vi "Tab.Set.vi"(8 "error in (no error)":errorcluster, 11 "State Variables":T1) -> (0 "error out":errorcluster, 3 "State Variables out":T1)   [LabVIEW 2015]
uses:
  Types/Main.StateVariables.ctl
  <vilib>/Utility/miscctls.llb/LVPositionTypeDef.ctl
  Types/Execute.UserEventRefs.ctl
  <vilib>/NI Veristand/Execution/Workspace/SystemStateRegEventRef.ctl
  <vilib>/NI Veristand/Execution/Workspace/Target State Info.ctl
  <vilib>/NI Veristand/Execution/Workspace/Target State.ctl
  <vilib>/NI Veristand/Execution/WaveformStreaming/Waveform Data Watcher Event Data (DBL).ctl
  <vilib>/NI Veristand/Execution/WaveformStreaming/WaveformStreamSpecification.ctl
  NationalInstruments.VeriStand.ClientAPI
  <vilib>/NI Veristand/Execution/Workspace/SystemStateEventRef.ctl
  <vilib>/NI Veristand/Execution/Workspace/WorkspaceAPI.ctl
  Types/UI.Object.ctl
  Types/Waveforms.Info.ctl
  <vilib>/NI Veristand/Execution/WaveformStreaming/Registered Waveform Streams Data Event Refnum (DBL).ctl
  <vilib>/NI Veristand/Execution/WaveformStreaming/WaveformDataWatcherDBL.ctl
  <vilib>/NI Veristand/Execution/WaveformStreaming/WaveformStreamingAPI.ctl
  <vilib>/Utility/miscctls.llb/LVRowAndColumnTypeDef.ctl
  <vilib>/NI Veristand/Execution/Workspace/NI_VS Workspace ExecutionAPI.lvlib
  <vilib>/NI Veristand/Execution/WaveformStreaming/NI_VS Waveform Streaming Interface.lvlib
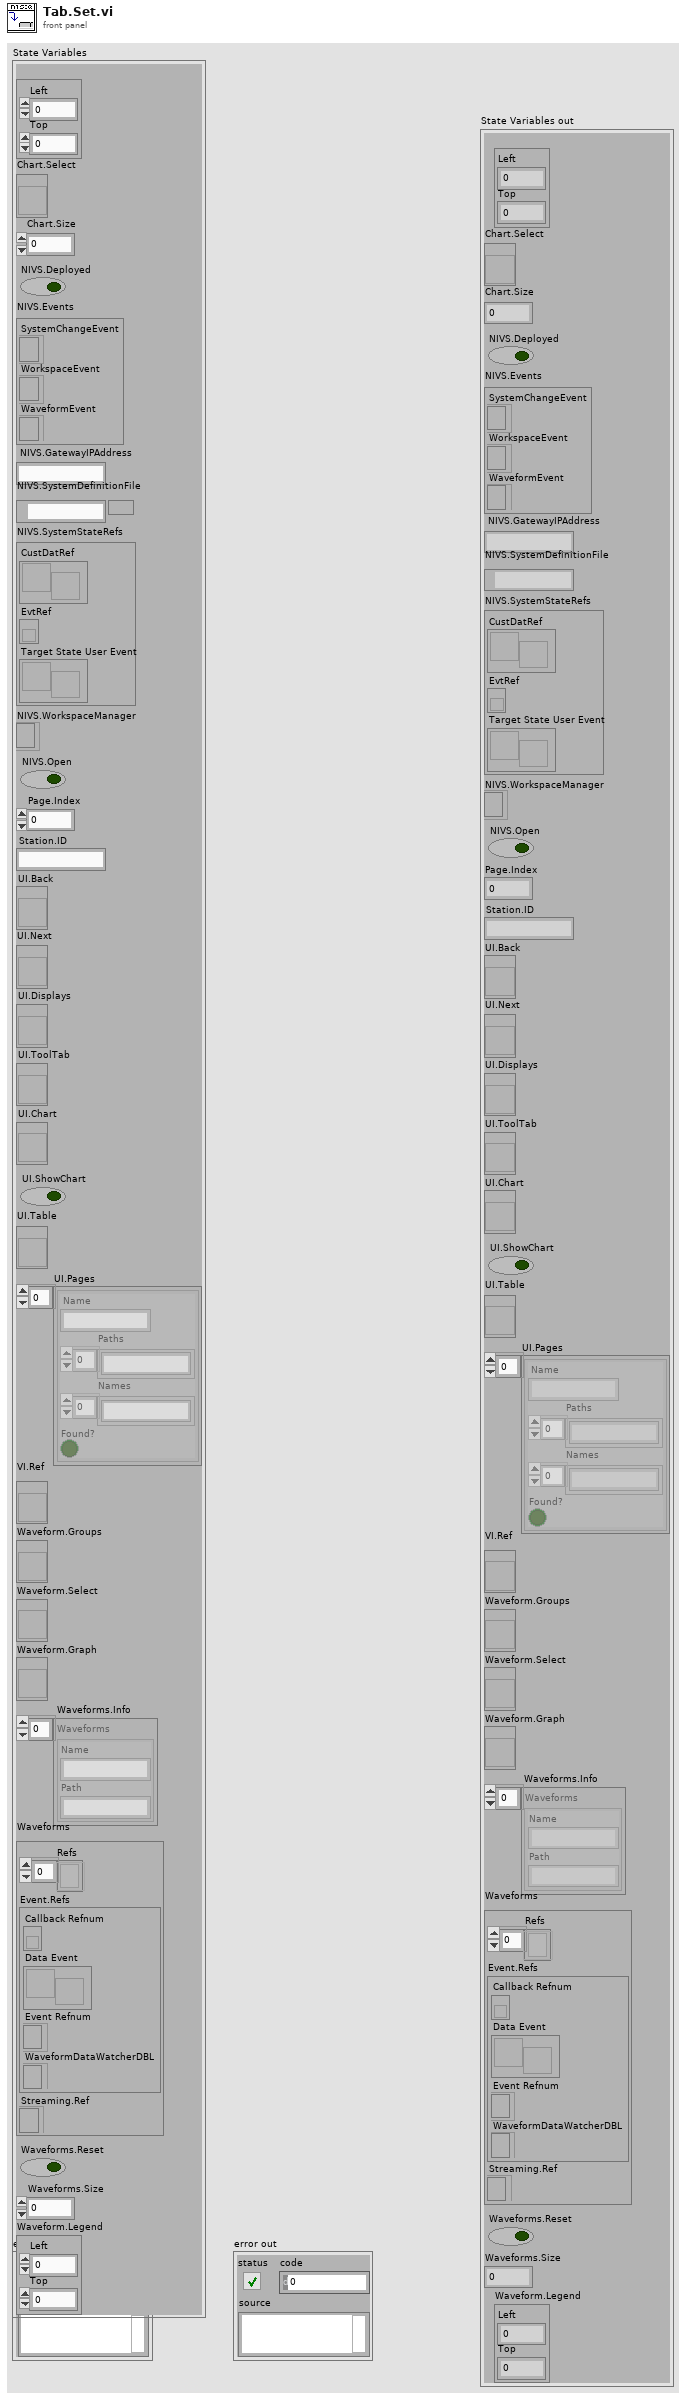
[diagram p1: front panel]
types:
  T1 = typedef "Main.StateVariables.ctl" = cluster{"Chart.Legend":T2, "Chart.Select":refnum<vi>, "Chart.Size":i32, "NIVS.Deployed":bool, "NIVS.Events":T3, "NIVS.GatewayIPAddress":string, "NIVS.SystemDefinitionFile":path, "NIVS.SystemStateRefs":T5, "NIVS.WorkspaceManager":T6, "NIVS.Open":bool, "Page.Index":u32, "Station.ID":string, "UI.Back":refnum<vi>, "UI.Next":refnum<vi>, "UI.Displays":refnum<vi>, "UI.ToolTab":refnum<vi>, "UI.Chart":refnum<vi>, "UI.ShowChart":bool, "UI.Table":refnum<vi>, "UI.Pages":T7[], "VI.Ref":refnum<vi>, "Waveform.Groups":refnum<vi>, "Waveform.Select":refnum<vi>, "Waveform.Graph":refnum<vi>, "Waveforms.Info":T8[], "Waveforms":cluster{"Refs":T9[], "Event.Refs":T10, "Streaming.Ref":T12}, "Waveforms.Reset":bool, "Waveforms.Size":i32, "Waveform.Legend":T2}
  T2 = typedef "LVPositionTypeDef.ctl" = cluster{"Left":i32, "Top":i32}
  T3 = typedef "Execute.UserEventRefs.ctl" = cluster{"SystemChangeEvent":T4, "WorkspaceEvent":refnum<event-registration>, "WaveformEvent":refnum<event-registration>}
  T4 = typedef "NI_VS Workspace ExecutionAPI.lvlib/SystemStateRegEventRef.ctl" = refnum<event-registration>
  T5 = typedef "NI_VS Workspace ExecutionAPI.lvlib/SystemStateEventRef.ctl" = cluster{"CustDatRef":refnum<user-event>, "EvtRef":refnum<k27>, "Target State User Event":refnum<user-event>}
  T6 = typedef "NI_VS Workspace ExecutionAPI.lvlib/WorkspaceAPI.ctl" = refnum<k24>
  T7 = typedef "UI.Object.ctl" = cluster{"Name":string, "Paths":string[], "Names":string[], "Found?":bool}
  T8 = typedef "Waveforms.Info.ctl" = cluster{"Name":string, "Path":string}
  T9 = typedef "NI_VS Waveform Streaming Interface.lvlib/WaveformStreamSpecification.ctl" = refnum<k24>
  T10 = typedef "NI_VS Waveform Streaming Interface.lvlib/Registered Waveform Streams Data Event Refnum (DBL).ctl" = cluster{"Callback Refnum":refnum<k27>, "Data Event":refnum<user-event>, "Event Refnum":refnum<event-registration>, "WaveformDataWatcherDBL":T11}
  T11 = typedef "NI_VS Waveform Streaming Interface.lvlib/WaveformDataWatcherDBL.ctl" = refnum<k24>
  T12 = typedef "NI_VS Waveform Streaming Interface.lvlib/WaveformStreamingAPI.ctl" = refnum<k24>
  T13 = typedef "LVRowAndColumnTypeDef.ctl" = cluster{"Row":i32, "Column":i32}
  T14 = typedef "LVBoundsTypeDef.ctl" = cluster{"Width":u32, "Height":u32}
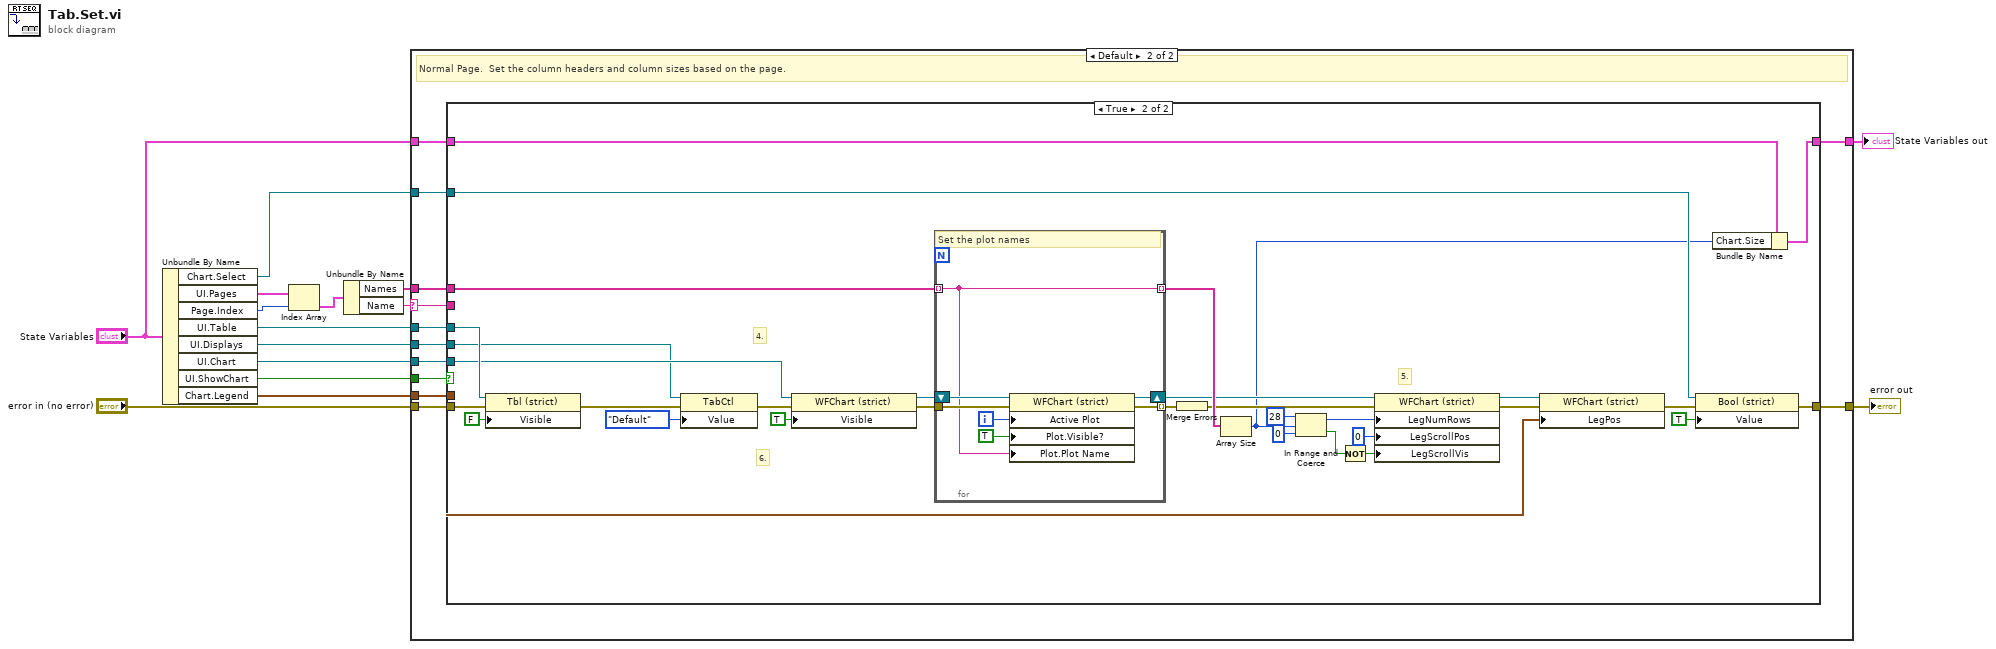
[diagram p0: block diagram]
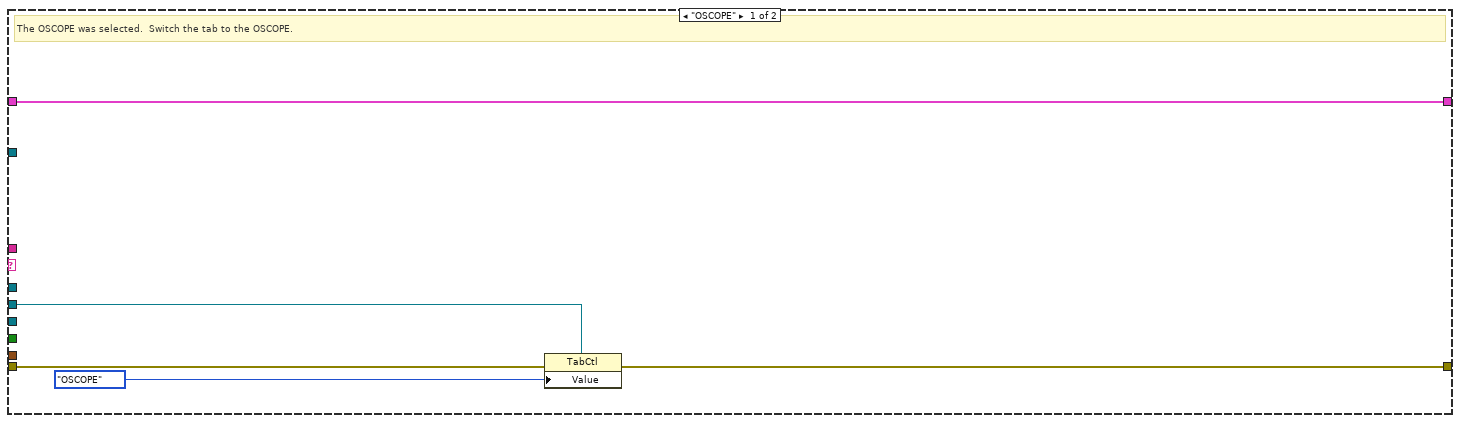
[diagram p2: hidden frame]
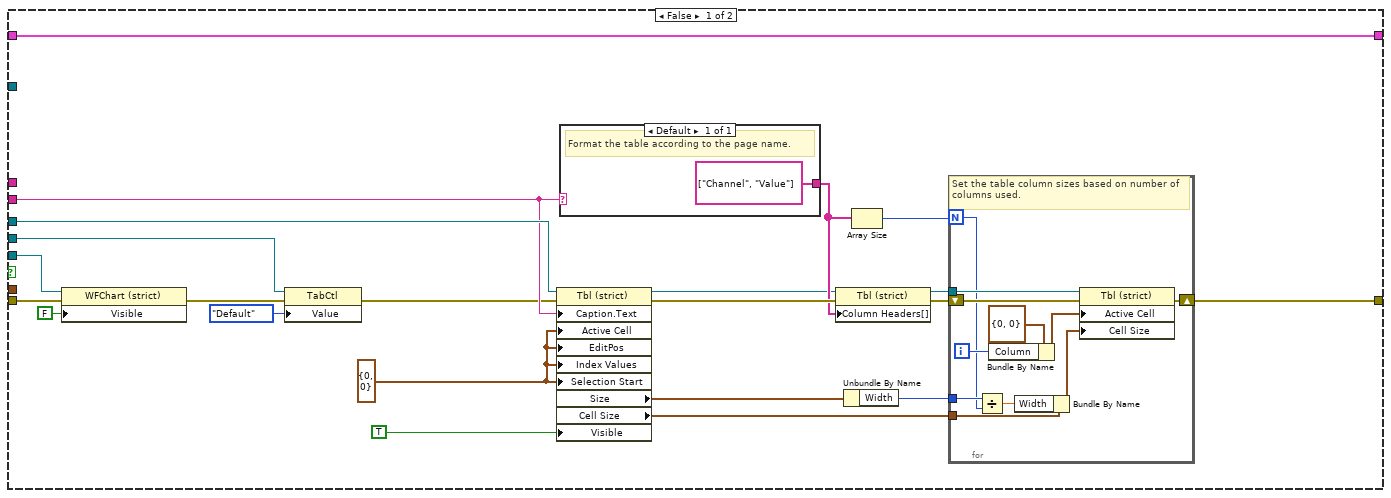
[diagram p3: hidden frame]
diagram:
  n1 = Unbundle By Name("State Variables") -> ("Chart.Select"=w3:refnum<vi>, "UI.Pages"=w8:T7[], "Page.Index"=w9:u32, "UI.Table"=w12:refnum<vi>, "UI.Displays"=w11:refnum<vi>, "UI.Chart"=w7:refnum<vi>, "UI.ShowChart"=w6:bool, "Chart.Legend"=w4:T2)
  n2 = Index Array(array=w8, index=w9) -> (element=w10:T7)
  n3 = Unbundle By Name(w10) -> ("Names"=w5:string[], "Name"=w13:string)
  n4 = case shown="Default" w13 {
    selector: w13 -> [_ w30]
    tunnel: w11 -> [w20 w27]
    tunnel: "error in (no error)" -> [w19 w28]
    tunnel: [w18 w31] -> w14
    tunnel: w12 -> [_ w32]
    tunnel: w7 -> [_ w29]
    tunnel: w6 -> [_ w26]
    tunnel: w5 -> [_ w25]
    tunnel: w4 -> [_ w24]
    tunnel: w3 -> [_ w23]
    tunnel: "State Variables" -> [w16 w22]
    tunnel: [w16 w21] -> w1
    frame "OSCOPE" {
      # "The OSCOPE was selected.  Switch the tab to the OSCOPE."
      n5 = property class="TabCtl"(reference=w20, error in=w19, "Value"=enum32{"Default", "OSCOPE"}."OSCOPE" ("Displays")) -> (error out=w18:errorcluster)  [unwired: 1 out]
    }
    frame Default {
      # "Normal Page.  Set the column headers and column sizes based on the page."
      n6 = case shown="True" w26 {
        tunnel: w32 -> [w54 w88]
        tunnel: [w49 w76] -> w31
        tunnel: w30 -> [w53 _]
        tunnel: w29 -> [w52 w83]
        tunnel: w28 -> [w51 w86]
        tunnel: w27 -> [w50 w67]
        tunnel: w25 -> [_ w89]
        tunnel: w24 -> [_ w78]
        tunnel: w23 -> [_ w75]
        tunnel: w22 -> [w33 w73]
        tunnel: [w33 w71] -> w21
        frame False {
          w46 = T13 {"Row"=0, "Column"=0} ("Selection Start")
          n7 = property class="WFChart (strict)"(reference=w52, error in=w51, "Visible"=FALSE) -> (error out=w36:errorcluster)  [unwired: 1 out]
          n8 = property class="TabCtl"(reference=w50, error in=w36, "Value"=enum32{"Default", "OSCOPE"}."Default" ("Displays")) -> (error out=w47:errorcluster)  [unwired: 1 out]
          n9 = property class="Tbl (strict)"(reference=w54, error in=w47, "Caption.Text"=w53, "Active Cell"=w46, "EditPos"=w46, "Index Values"=w46, "Selection Start"=w46, "Visible"=TRUE) -> (reference out=w38:refnum<vi>, error out=w45:errorcluster, "Size"=w42:T14, "Cell Size"=w40:T14)
          n10 = case shown="Default" w53 {
            tunnel: [string[] ["Channel", "Value"]] -> w39
            frame Default {
              # "Format the table according to the page name."
            }
          }
          n11 = property class="Tbl (strict)"(reference=w38, error in=w45, "Column Headers[]"=w39) -> (reference out=w44:refnum<vi>, error out=w43:errorcluster)
          n12 = Unbundle By Name(w42) -> ("Width"=w41:u32)
          n13 = Array Size(array=w39) -> (size(s)=w37:i32)
          n14 = for {
            N: w37 -> [w56]
            tunnel: w44 -> [w66]
            shift-right: [w64] -> w49
            shift-left: w43 -> [w65]
            tunnel: w41 -> [w62]
            tunnel: w40 -> [w63]
            i -> [w58]
            # "Set the table column sizes based on number of columns used."
            n15 = Divide(x=w62, y=w56) -> (x/y=w57:dbl)
            n16 = Bundle By Name(cluster=T13 {"Row"=0, "Column"=0} ("Active Cell:Active Cell"), "Column"=w58) -> (w59:T13)
            n17 = Bundle By Name(cluster=w63, "Width"=w57) -> (w61:T14)
            n18 = property class="Tbl (strict)"(reference=w66, error in=w65, "Active Cell"=w59, "Cell Size"=w61) -> (error out=w64:errorcluster)  [unwired: 1 out]
          }
        }
        frame True {
          # "4."
          # "6."
          # "5."
          n19 = property class="Tbl (strict)"(reference=w88, error in=w86, "Visible"=FALSE) -> (error out=w69:errorcluster)  [unwired: 1 out]
          n20 = property class="TabCtl"(reference=w67, error in=w69, "Value"=enum32{"Default", "OSCOPE"}."Default" ("Displays")) -> (error out=w68:errorcluster)  [unwired: 1 out]
          n21 = property class="WFChart (strict)"(reference=w83, error in=w68, "Visible"=TRUE) -> (reference out=w82:refnum<vi>, error out=w84:errorcluster)
          n22 = for {
            tunnel: w89 -> [w99] mode=indexing
            tunnel: [w99] -> w97 mode=indexing
            shift-right: [w101] -> w93
            shift-left: w82 -> [w105]
            tunnel: w84 -> [w104]
            tunnel: [w103] -> w98 mode=indexing
            i -> [w102]
            # "Set the plot names"
            n23 = property class="WFChart (strict)"(reference=w105, error in=w104, "Active Plot"=w102, "Plot.Visible?"=TRUE ("Plot.Visible"), "Plot.Plot Name"=w99) -> (reference out=w101:refnum<vi>, error out=w103:errorcluster)
          }
          n24 = Merge Errors(w98) -> (w85:errorcluster)
          n25 = Array Size(array=w97) -> (size(s)=w72:i32)
          n26 = In Range and Coerce(upper limit=28, x=w72, lower limit=0) -> (coerced(x)=w94:i32, In Range?=w91:bool)
          n27 = Not(x=w91) -> (.not. x?=w90:bool)
          n28 = property class="WFChart (strict)"(reference=w93, error in=w85, "LegNumRows"=w94, "LegScrollPos"=u32 0 ("Legend:Scroll Position"), "LegScrollVis"=w90) -> (reference out=w79:refnum<vi>, error out=w80:errorcluster)
          n29 = property class="WFChart (strict)"(reference=w79, error in=w80, "LegPos"=w78) -> (error out=w77:errorcluster)  [unwired: 1 out]
          n30 = property class="Bool (strict)"(reference=w75, error in=w77, "Value"=TRUE) -> (error out=w76:errorcluster)  [unwired: 1 out]
          n31 = Bundle By Name(cluster=w73, "Chart.Size"=w72) -> (w71:T1)
        }
      }
    }
  }
  "error out" <- w14
  "State Variables out" <- w1
